vi "SetSupplyVoltage.vi"(10 "Voltage":u8(ring) items=["1.2"=0, "1.5"=4, "1.8"=1, "2.1"=5, "2.4"=6, "2.7"=7, "3,0"=8, "3.3"=2, "3.6"=9, "4.5"=10, "5.0"=3, "5.5"=11], 11 "Port":enum8{"ONE", "TWO"}(ring)) -> (3 "ByteArrayToSend":u8[](array[numeric]) format="%x")   [LabVIEW 2019]
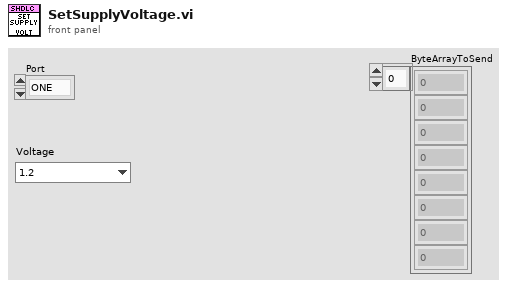
[diagram p1: front panel]
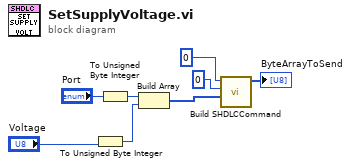
[diagram p0: block diagram]
diagram:
  n1 = To Unsigned Byte Integer(number="Voltage") -> (unsigned 8bit integer=w2:u8)
  n2 = To Unsigned Byte Integer(number="Port") -> (unsigned 8bit integer=w5:u8)
  n3 = Build Array(w5, w2) -> (w4:u8[])
  n4 = call "Build SHDLCCommand.vi"("Data"=w4, "CommandID"=u8 0, "SlaveAdress"=u8 0) -> ("ByteArrayToSend"=→"ByteArrayToSend":u8[])  [unwired: 8 in]
